vi "niRFUtil CONV 1 Ohm Voltage to 1 Ohm Watt (real scalar).vi"(7 "Real Scalar (V)":sgl format="%.2f") -> (8 "Real Scalar (W)":sgl format="%.2f")   [LabVIEW 2015, in "niRFUtil.lvlib"]
doc: "(c) Copyright 2006, National Instruments, Inc. This VI may not be duplicated, sold, or distributed without written consent from National Instruments."
uses:
  niRFUtil.lvlib
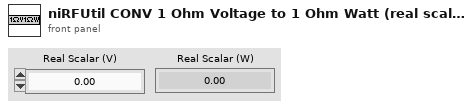
[diagram p1: front panel]
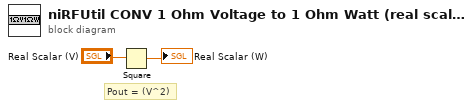
[diagram p0: block diagram]
diagram:
  # "Pout = (V^2)"
  n1 = Square(x="Real Scalar (V)") -> (x^2=→"Real Scalar (W)":sgl)
